vi "Get Filtered Sets.vi"(5 "Device Class":string, 6 "Product ID":i32 format="%.0x", 7 "Operating System":string, 8 "error in (no error)":errorcluster, 10 "Item Types (all visible)":T1 items=["all visible", "all including hidden", "standard only", "startup only"], 11 "Repository in (RT Images)":path) -> (0 "error out":errorcluster, 2 "Software Sets":T2[](array[typedef]) {"information"."component type" items=["standard", "hidden", "system", "unknown", "startup", "image", "essential"]; "items"."component type" items=["standard", "hidden", "system", "unknown", "startup", "image", "essential"]; "add-ons"."component type" items=["standard", "hidden", "system", "unknown", "startup", "image", "essential"]}, 3 "Repository out":path)   [LabVIEW 2020, in "nisyscfg.lvlib"]
doc: "Retrieves a list of software sets on the local system that are available for installation to the specified target. Not all Real-Time systems support the installation of software sets."
uses:
  <vilib>/nisyscfg/nisyscfg.lvlib
  <vilib>/nisyscfg/Software Set 1.2.ctl
  <vilib>/nisyscfg/Software 1.2.ctl
  <vilib>/nisyscfg/Component Type.ctl
  <vilib>/nisyscfg/Component Types.ctl
  <resource>/objmgr/nisysapi.rc
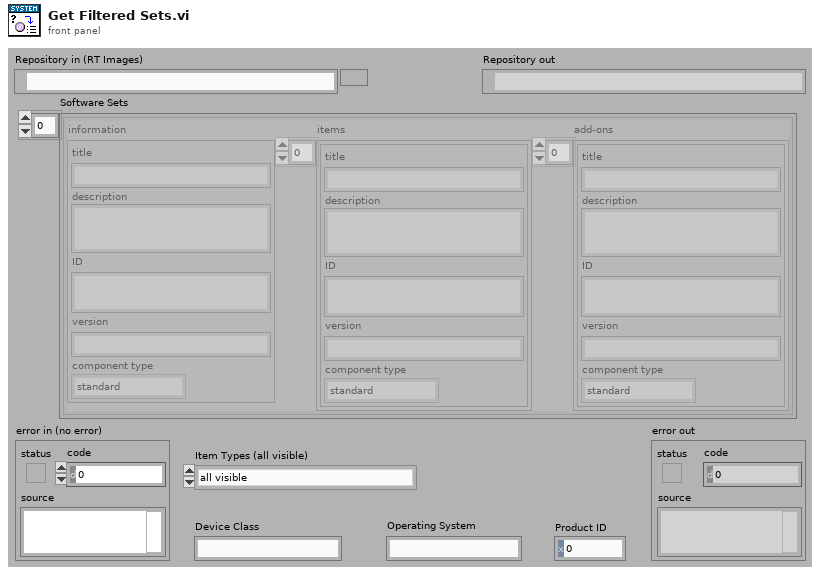
[diagram p1: front panel]
types:
  T1 = typedef "nisyscfg.lvlib/Component Types.ctl" = u32
  T2 = typedef "nisyscfg.lvlib/Software Set 1.2.ctl" = cluster{"information":T3, "items":T3[], "add-ons":T3[]}
  T3 = typedef "nisyscfg.lvlib/Software 1.2.ctl" = cluster{"title":string, "description":string, "ID":string, "version":string, "component type":T4}
  T4 = typedef "nisyscfg.lvlib/Component Type.ctl" = u32
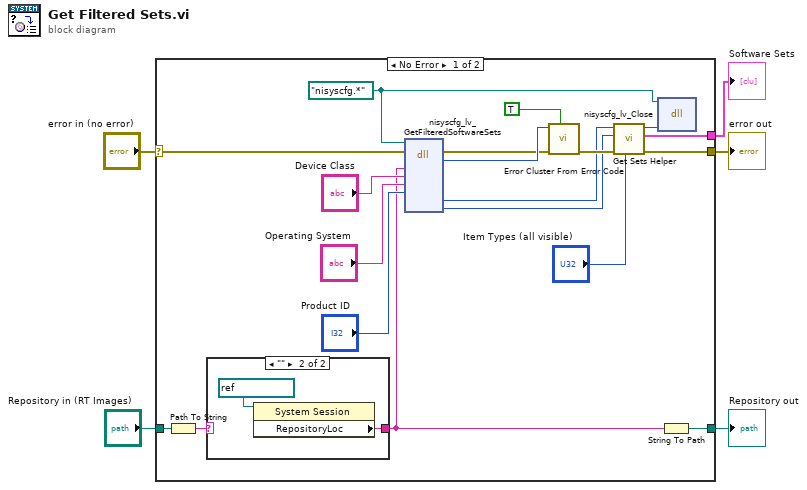
[diagram p0: block diagram]
diagram:
  n1 = case shown="No Error" "error in (no error)" {
    selector: "error in (no error)" -> [w22 w29]
    tunnel: [w16 w29] -> w5
    tunnel: "Repository in (RT Images)" -> [w9 w28]
    tunnel: [w17 _] -> w2
    tunnel: [w6 w28] -> w1
    frame No Error {
      w14 = path "nisyscfg.*" ("path in")
      n2 = Path To String(path=w9) -> (string=w8:string)
      n3 = case shown="\"\"" w8 {
        selector: w8 -> [w25 _]
        tunnel: [w25 w27] -> w7
        frame Default {
        }
        frame "" {
          n4 = property class="System Session"(reference=refnum<k21> "localhost" ("System Configuration")) -> ("RepositoryLoc"=w27:string)  [unwired: 1 in, 2 out]
        }
      }
      n5 = dll-call lib="nisyscfg.*" fn="nisyscfg_lv_GetFilteredSoftwareSets" label="GetFilteredSoftwareSets"(path in=w14, error in=w22, "repository"=w7, "deviceClass"="Device Class", "operatingSystem"="Operating System", "productID"="Product ID") -> (error out=w23:errorcluster, "result"=w24:i32, "softwareSets"=w11:u64, "numSets"=w12:i32)  [unwired: 7 in, 1 out]
      n6 = call <vilib>:"Error Cluster From Error Code.vi"("show call chain? (False)"=TRUE, "error in (no error)"=w23, "error code (0)"=w24) -> ("error out"=w13:errorcluster)  [unwired: 6 in]
      n7 = call <vilib>:"Get Sets Helper.vi"("Item Types (all visible)"="Item Types (all visible)", "error in (no error)"=w13, "Number of Elements"=w12, "Enumerator in"=w11) -> ("error out"=w16:errorcluster, "Software Sets"=w17:T2[], "Enumerator out"=w15:u64)  [unwired: 5 in]
      n8 = dll-call lib="nisyscfg.*" fn="nisyscfg_lv_Close" label="Close"(path in=w14, "expertsEnum"=w15) -> ()  [unwired: 3 in, 3 out]
      n9 = String To Path(string=w7) -> (path=w6:path)
    }
    frame Error {
    }
  }
  "error out" <- w5
  "Software Sets" <- w2
  "Repository out" <- w1
